vi "Get Steering Motor Angle Setpoint.vi"(8 "error in (no error)":errorcluster, 11 "wheel in":refnum<class "NI_Robotics_Wheel.lvclass">) -> (0 "error out":errorcluster, 1 "failed?":bool, 2 "ccw motor angle setpoint (rad)":dbl, 3 "wheel out":refnum<class "NI_Robotics_Wheel.lvclass">)   [LabVIEW 2017, in "NI_Robotics_Wheel.lvclass"]
uses:
  <vilib>/robotics/Steering/Wheel/NI_Robotics_Wheel.lvclass
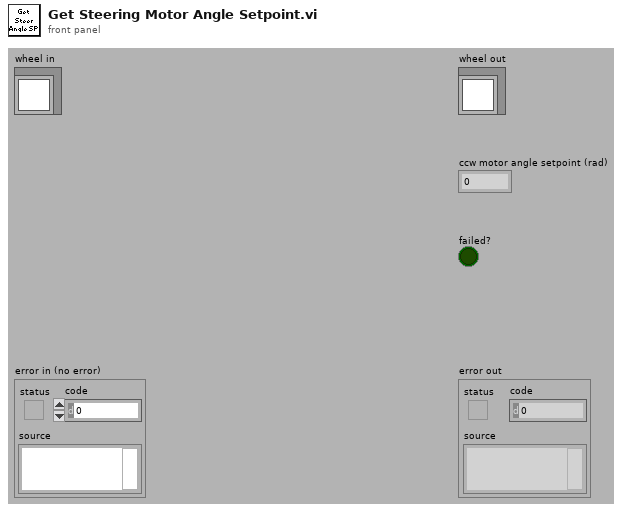
[diagram p1: front panel]
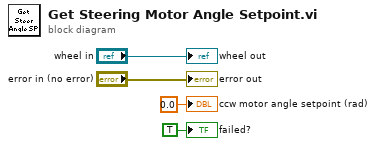
[diagram p0: block diagram]
diagram:
  "error out" <- "error in (no error)"
  "wheel out" <- "wheel in"
  "ccw motor angle setpoint (rad)" <- 0.0 ("ccw motor angle")
  "failed?" <- TRUE ("failed?")
